vi "pathOperations.vi"() -> ()   [LabVIEW 2014]
panel:
  out "File I/O Error State":errorcluster
  in  "File Access Specifier":enum16{"read/write", "read-only", "write-only"}(ring)
  in  "File Operation Specifier":T1(ring)
  in  "File Name":string
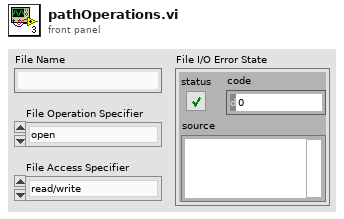
[diagram p1: front panel]
types:
  T1 = enum16{"open", "replace", "create", "open or create", "replace or create", "replace or create with confirmation"}
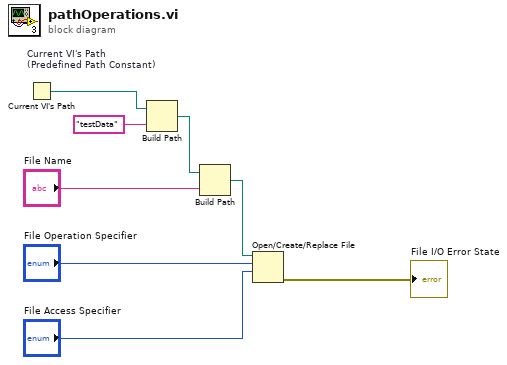
[diagram p0: block diagram]
diagram:
  n1 = Current VI's Path "Current VI's Path\n(Predefined Path Constant)"() -> (path=w8:path)
  n2 = Build Path(base path=w8, name or relative path="testData") -> (appended path=w6:path)
  n3 = Build Path(base path=w6, name or relative path="File Name") -> (appended path=w4:path)
  n4 = Open/Create/Replace File(file path (use dialog)=w4, operation (0:open)="File Operation Specifier", access (0:read/write)="File Access Specifier") -> (error out=→"File I/O Error State":errorcluster)  [unwired: 3 in, 2 out]
